vi "non_FPGA_VI_v2.vi"() -> ()   [LabVIEW 2020]
uses:
  c5c29772-c0b0-45e0-ac49-cc5077cfdad3.vi
  <vilib>/Array/Sort 2D Array - Pop Stack.vi
  <vilib>/Array/Sort 2D Array - Push Stack.vi
  c5c29772-c0b0-45e0-ac49-cc5077cfdad3.vi/269d4b3b-47f5-49e3-8884-44851e4dd9d5.vi
  c5c29772-c0b0-45e0-ac49-cc5077cfdad3.vi/6d99389c-673d-4efb-bf33-19b32bcf4cf8.vi
  <vilib>/Analysis/NI_AALBase.lvlib
panel:
  out "sorted array":sgl[](graph)
  out "sorted array index":i32[](array[numeric])
  out "sorted array img":sgl[](array[numeric])
  out "sorted array real":sgl[](array[numeric])
  out "sorted 2D array":sgl[][](array[numeric])
  out "appended array":sgl[][](array[numeric])
  out "sorted array":sgl[](array[numeric])
  out "uniform white noise":sgl[](array[numeric])
  out "array input":sgl[](graph)
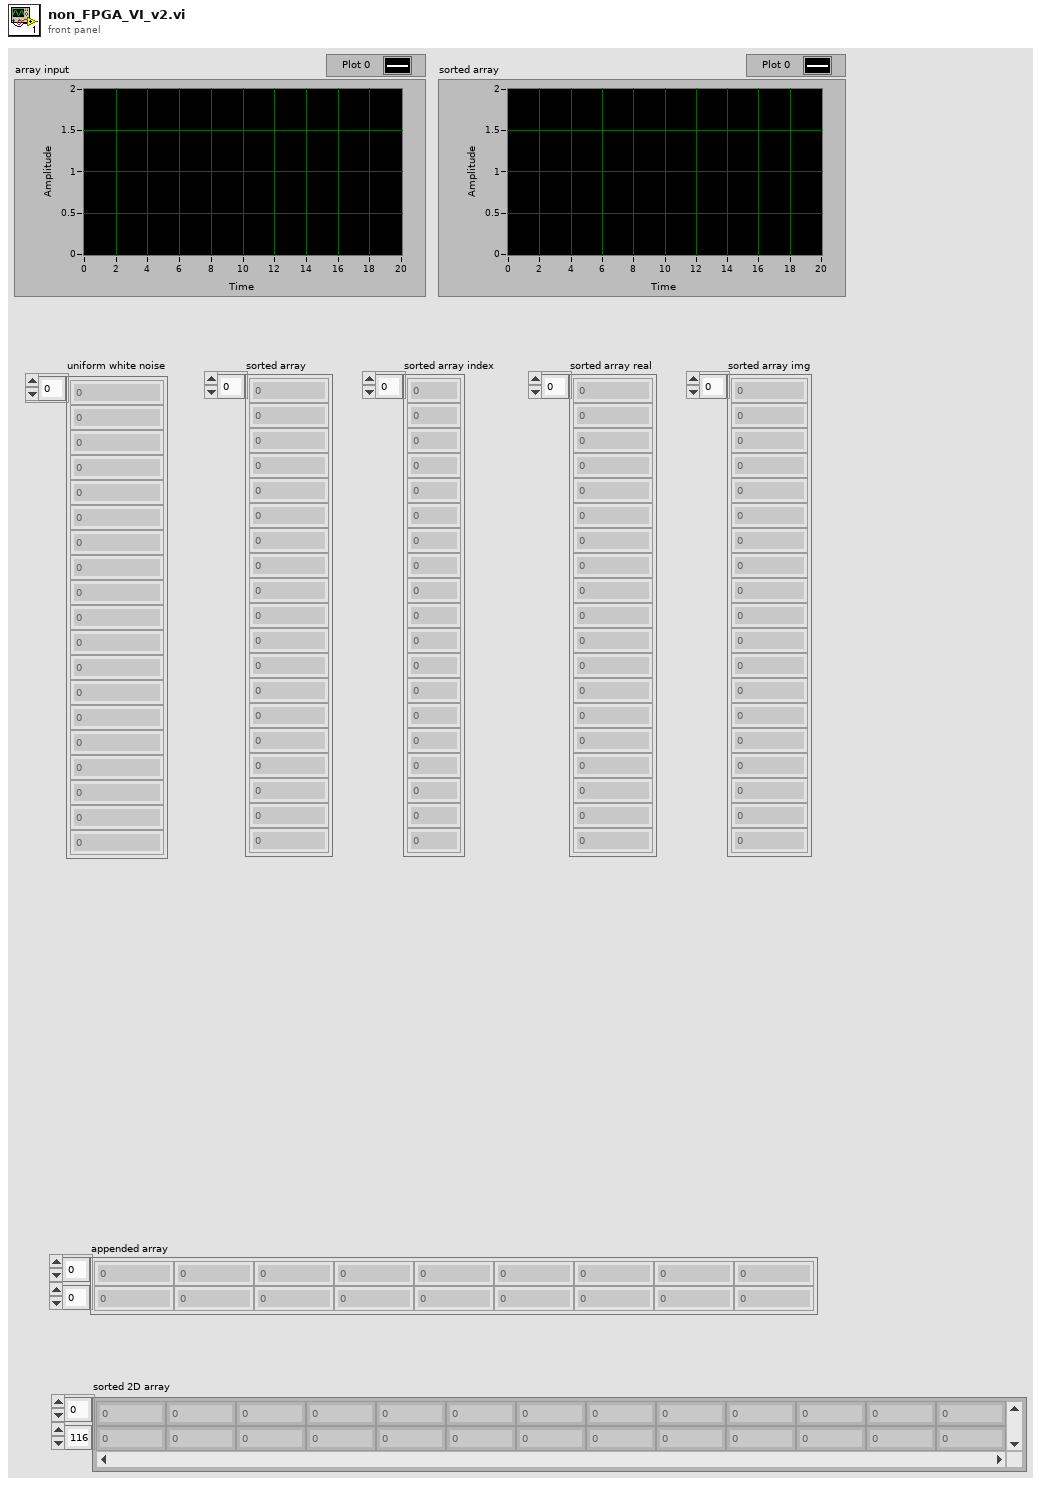
[diagram p1: front panel]
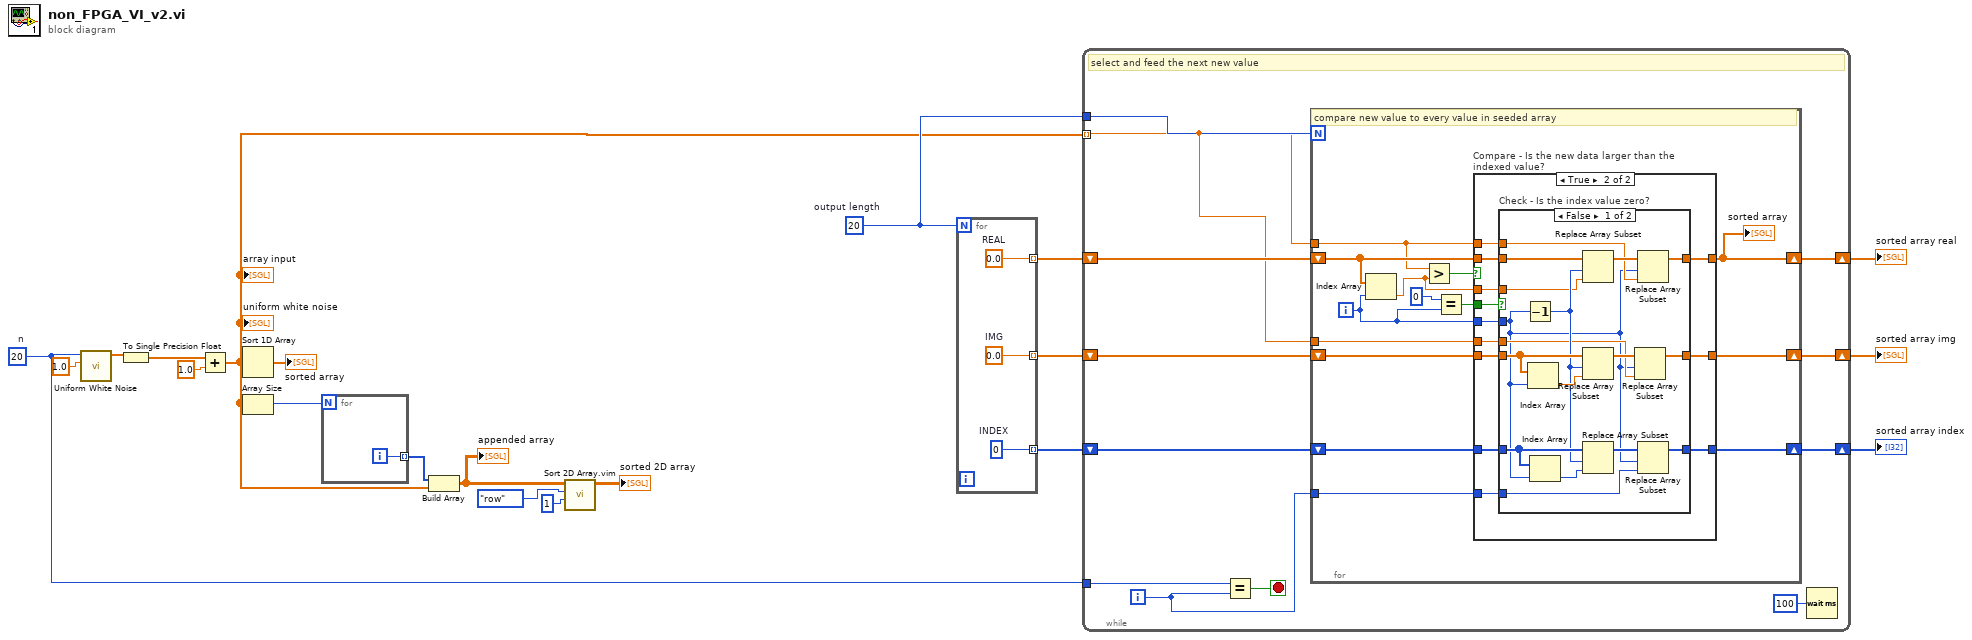
[diagram p0: block diagram]
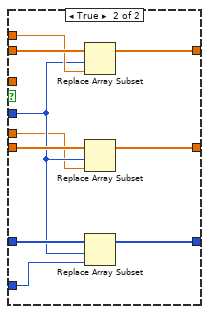
[diagram p3: hidden frame]
diagram:
  w9 = 20  # output length
  w10 = 20  # n
  n1 = call <vilib>:"Uniform White Noise.vi"("amplitude"=1.0, "samples"=w10) -> ("uniform white noise"=w3:dbl[])  [unwired: 8 in, 1 out]
  n2 = To Single Precision Float(number=w3) -> (single precision float=w2:sgl[])
  n3 = Add(x=w2, y=sgl 1.0 ("amplitude")) -> (x+y=w1:sgl[])
  "array input" <- w1
  "uniform white noise" <- w1
  n4 = Sort 1D Array(array=w1) -> (sorted array=→"sorted array":sgl[])
  n5 = Array Size(array=w1) -> (size(s)=w17:i32)
  n6 = for {
    N: w17 -> [_]
    tunnel: [w21] -> w16 mode=indexing
    i -> [w21]
  }
  n7 = Build Array(w16, w1) -> (w7:sgl[][])
  "appended array" <- w7
  n8 = call "Sort 2D Array.vim"("index"=1, "dimension to index (column)"=enum16{"column", "row"}."row", "2D array"=w7) -> ("sorted 2D array"=→"sorted 2D array":sgl[][])  [unwired: 7 in, 1 out]
  n9 = for {
    N: w9 -> [_]
    tunnel: [w24] -> w14 mode=indexing
    tunnel: [w23] -> w15 mode=indexing
    tunnel: [w22] -> w13 mode=indexing
    w22 = sgl 0.0  # IMG
    w23 = 0  # INDEX
    w24 = sgl 0.0  # REAL
  }
  n10 = while {
    shift-right: [w27] -> w8
    shift-left: w14 -> [w36]
    shift-right: [w35] -> w12
    shift-left: w15 -> [w34]
    tunnel: w10 -> [w32]
    shift-right: [w30] -> w11
    shift-left: w13 -> [w29]
    tunnel: w1 -> [w25] mode=indexing
    tunnel: w9 -> [w28]
    i -> [w33]
    stop <- w31 stop-if-true
    # "select and feed the next new value"
    n11 = Equal?(x=w32, y=w33) -> (x = y?=w31:bool)
    n12 = for {
      N: w28 -> [_]
      tunnel: w25 -> [w48]
      shift-right: [w47] -> w27
      shift-left: w36 -> [w49]
      tunnel: w33 -> [w45]
      shift-right: [w43] -> w35
      shift-left: w34 -> [w44]
      shift-right: [w40] -> w30
      shift-left: w29 -> [w39]
      tunnel: w25 -> [w38]
      i -> [w46]
      # "compare new value to every value in seeded array"
      n13 = Index Array(array=w49, index=w46) -> (element=w37:sgl)
      n14 = Greater?(x=w48, y=w37) -> (0:w50:bool)
      n15 = Equal?(x=0, y=w46) -> (x = y?=w41:bool)
      n16 = case "Compare - Is the new data larger than the indexed value?" shown="True" w50 {
        tunnel: w49 -> [w53 w64]
        tunnel: w41 -> [_ w65]
        tunnel: w48 -> [_ w63]
        tunnel: w46 -> [_ w62]
        tunnel: [w53 w61] -> w47
        tunnel: w45 -> [_ w60]
        tunnel: w44 -> [w52 w59]
        tunnel: [w52 w58] -> w43
        tunnel: [w51 w57] -> w40
        tunnel: w39 -> [w51 w56]
        tunnel: w38 -> [_ w55]
        tunnel: w37 -> [_ w54]
        frame False {
        }
        frame True {
          n17 = case "Check - Is the index value zero?" shown="False" w65 {
            tunnel: w64 -> [w82 w92]
            tunnel: w63 -> [w80 w91]
            tunnel: w62 -> [w67 w85]
            tunnel: [w79 w90] -> w61
            tunnel: w60 -> [w74 w89]
            tunnel: w59 -> [w76 w88]
            tunnel: [w75 w87] -> w58
            tunnel: [w69 w83] -> w57
            tunnel: w56 -> [w73 w86]
            tunnel: w55 -> [w68 w84]
            tunnel: w54 -> [w66 _]
            frame False {
              n18 = Decrement(x=w67) -> (x-1=w71:i32)
              n19 = Index Array(array=w73, index=w67) -> (element=w72:sgl)
              n20 = Index Array(array=w76, index=w67) -> (element=w78:i32)
              n21 = Replace Array Subset(array=w82, new element=w66, index=w71) -> (w81:sgl[])
              n22 = Replace Array Subset(array=w73, new element=w72, index=w71) -> (w70:sgl[])
              n23 = Replace Array Subset(array=w76, new element=w78, index=w71) -> (w77:i32[])
              n24 = Replace Array Subset(array=w70, new element=w68, index=w67) -> (w69:sgl[])
              n25 = Replace Array Subset(array=w81, new element=w80, index=w67) -> (w79:sgl[])
              n26 = Replace Array Subset(array=w77, new element=w74, index=w67) -> (w75:i32[])
            }
            frame True {
              n27 = Replace Array Subset(array=w92, new element=w91, index=w85) -> (w90:sgl[])
              n28 = Replace Array Subset(array=w86, new element=w84, index=w85) -> (w83:sgl[])
              n29 = Replace Array Subset(array=w88, new element=w89, index=w85) -> (w87:i32[])
            }
          }
        }
      }
      "sorted array" <- w47
    }
    n30 = Wait (ms)(milliseconds to wait=u32 100) -> ()  [unwired: 1 out]
  }
  "sorted array real" <- w8
  "sorted array img" <- w11
  "sorted array index" <- w12
